vi "Write closeConnection.vi"(8 "error in (no error)":errorcluster, 10 "closeConnection":bool, 11 "STOMP in":refnum<class "STOMP.lvclass">) -> (0 "error out":errorcluster, 3 "STOMP out":refnum<class "STOMP.lvclass">)   [LabVIEW 2017, in "STOMP.lvclass"]
uses:
  STOMP.lvclass
  STOMP.lvclass/STOMP.ctl
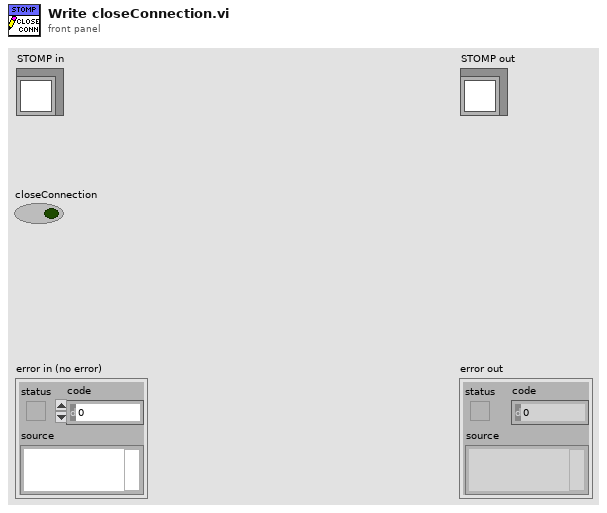
[diagram p1: front panel]
types:
  T1 = typedef "LabVIEW STOMP.lvlib/STOMP.lvclass/ObjectAttributes.ctl" = cluster{"address":string, "port":u16, "ConnectionRef":refnum<k5>, "messageQueue":refnum<queue>, "receiptQueue":refnum<queue>, "errorQueue":refnum<queue>, "sendQueue":refnum<queue>, "currentReceiptNumber":u64, "currentSubscriptionId":u64, "closeConnection":bool, "activeSubscriptions":T2[]}
  T2 = typedef "Type_ActiveSubscription.ctl" = cluster{"id":u64, "receipt":bool, "Destination":string, "ack":T3, "headers":T4[]}
  T3 = typedef "Type_AckHeader.ctl" = enum16{"auto", "client", "client-individual"}
  T4 = typedef "LabVIEW STOMP.lvlib/STOMP.lvclass/Type_FrameHeader.ctl" = cluster{"Header":string, "Value":string}
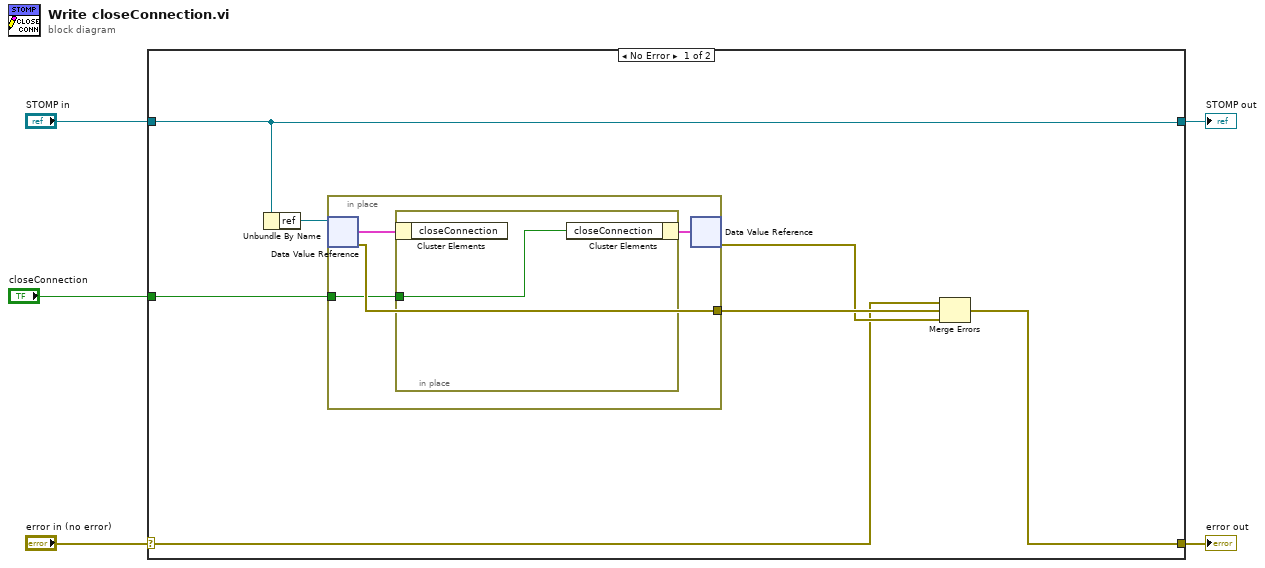
[diagram p0: block diagram]
diagram:
  n1 = case shown="No Error" "error in (no error)" {
    selector: "error in (no error)" -> [w7 w18]
    tunnel: [w6 w18] -> w4
    tunnel: [w10 w19] -> w2
    tunnel: "STOMP in" -> [w10 w19]
    tunnel: "closeConnection" -> [w11 _]
    frame No Error {
      n2 = Unbundle By Name(w10) -> ("ref"=w12:refnum<data-value>)
      n3 = in-place {
        in-place-border: w11 -> [w14]
        in-place-border: [w16] -> w9
        n4 = in-place-dvr #1(w12) -> (w15:T1, w16:errorcluster)
        n5 = in-place {
          in-place-border: w14 -> [w17]
          n6 = in-place-cluster #2(w15) -> ()  [unwired: 1 out]
          n7 = in-place-cluster #2("closeConnection"=w17) -> (w13:T1)
        }
        n8 = in-place-dvr #1(w13) -> (w8:errorcluster)  [unwired: 1 out]
      }
      n9 = Merge Errors(w7, w9, w8) -> (w6:errorcluster)
    }
    frame Error {
    }
  }
  "error out" <- w4
  "STOMP out" <- w2
